vi "Launch.vi"(5 "window position":cluster{"Left":i16, "Top":i16}, 7 "options":T1, 8 "error in (no error)":errorcluster, 11 "Thread in":refnum<class "Thread.lvclass">) -> (0 "error out":errorcluster, 3 "Thread out":refnum<class "Thread.lvclass">)   [LabVIEW 2017, in "DSF Core.lvlib" / "Thread.lvclass"]
uses:
  Thread.lvclass
  DSF Thread Options.ctl
  Thread.lvclass/Thread.ctl
  Top.vi
  DSF Core.lvlib
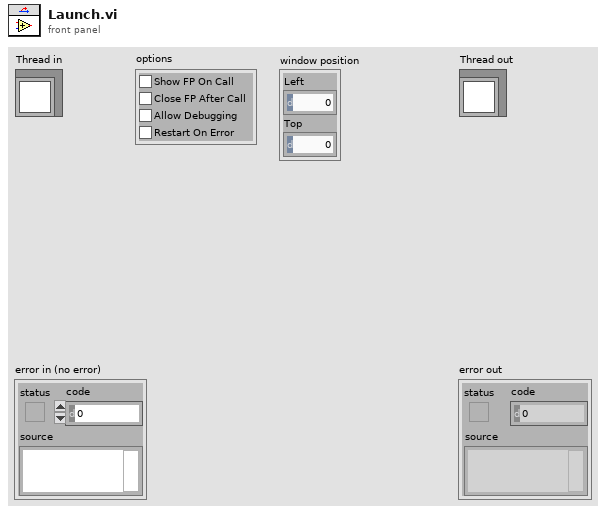
[diagram p1: front panel]
types:
  T1 = typedef "DSF Core.lvlib/DSF Thread Options.ctl" = cluster{"Show FP On Call":bool, "Close FP After Call":bool, "Allow Debugging":bool, "Restart On Error":bool}
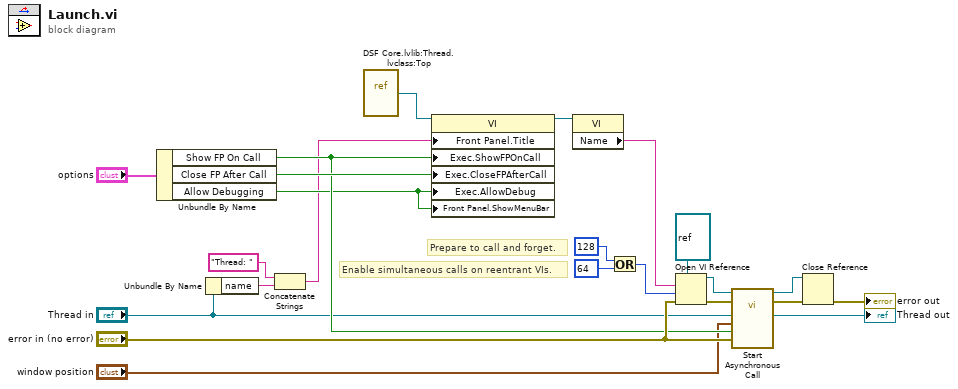
[diagram p0: block diagram]
diagram:
  # "Prepare to call and forget."
  # "Enable simultaneous calls on reentrant VIs."
  n1 = Unbundle By Name("options") -> ("Show FP On Call"=w5:bool, "Close FP After Call"=w14:bool, "Allow Debugging"=w4:bool)
  n2 = Unbundle By Name("Thread in") -> ("name"=w12:string)
  n3 = Concatenate Strings("Thread: " ("string"), w12) -> (w3:string)
  n4 = vi-ref "DSF Core.lvlib:Thread.lvclass:Top.vi"() -> (w11:refnum<vi>)
  n5 = property class="VI"(reference=w11, "Front Panel.Title"=w3, "Exec.ShowFPOnCall"=w5, "Exec.CloseFPAfterCall"=w14, "Exec.AllowDebug"=w4, "Front Panel.ShowMenuBar"=w4) -> (reference out=w16:refnum<vi>)  [unwired: 1 in, 1 out]
  n6 = property class="VI"(reference=w16) -> ("Name"=w6:string)  [unwired: 1 in, 2 out]
  n7 = Or(x=128 ("options"), y=64 ("options")) -> (x .or. y?=w18:i32)
  n8 = Open VI Reference(type specifier VI Refnum (for type only)=refnum<vi> refnum, vi path=w6, options=w18, error in (no error)="error in (no error)") -> (vi reference=w9:refnum<vi>, error out=w10:errorcluster)  [unwired: 2 in]
  n9 = call-by-ref "Start Asynchronous Call"(reference=w9, error in=w10, 8:"error in (no error)"="error in (no error)", "reposition window"=w5, "window position"="window position", "Thread in"="Thread in") -> (reference out=w7:refnum<vi>, error out=w8:errorcluster)  [unwired: 6 in, 2 out]
  n10 = Close Reference(reference=w7, error in (no error)=w8) -> (error out=→"error out":errorcluster)
  "Thread out" <- "Thread in"
